vi "RichToFlatnixnet_grpc_EnetFrameRequest.vi"(5 "OutputClusterType":T1, 11 "InputCluster":T4) -> (3 "OutputCluster":T1)   [LabVIEW 2025, in "grpc-xnet_client.lvlib"]
uses:
  grpc-xnet_client.lvlib
  nixnet_grpc_EnetFrameRequest.ctl
  nixnet_grpc_EnetFrameRequest_type_enum/nixnet_grpc_EnetFrameRequest_type_enum.lvclass
  nixnet_grpc_EnetFlags.ctl
  nixnet_grpc_EnetFrameRequest_Flat.ctl
  nixnet_grpc_EnetFrameType.ctl
  nixnet_grpc_EnetFrameRequest_type_enum/nixnet_grpc_EnetFrameRequest_type_enum.lvclass/nixnet_grpc_EnetFrameRequest_type_enum.ctl
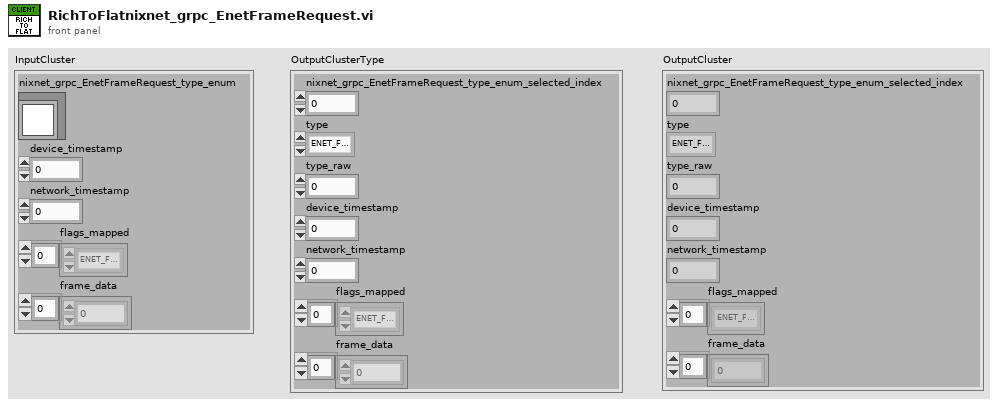
[diagram p1: front panel]
types:
  T1 = typedef "grpc-xnet_client.lvlib/nixnet_grpc_EnetFrameRequest_Flat.ctl" = cluster{"nixnet_grpc_EnetFrameRequest_type_enum_selected_index":i32, "type":T2, "type_raw":u32, "device_timestamp":u64, "network_timestamp":u64, "flags_mapped":T3[], "frame_data":u8[]}
  T2 = typedef "grpc-xnet_client.lvlib/nixnet_grpc_EnetFrameType.ctl" = enum32{"ENET_FRAME_TYPE_DATA", "ENET_FRAME_TYPE_DELAY", "ENET_FRAME_TYPE_FUTURE_TIME_WAIT"}
  T3 = typedef "grpc-xnet_client.lvlib/nixnet_grpc_EnetFlags.ctl" = enum32{"ENET_FLAGS_UNSPECIFIED", "ENET_FLAGS_TRANSMIT", "ENET_FLAGS_RECEIVE", "ENET_FLAGS_NETWORK_SYNCED", "ENET_FLAGS_ERROR"}
  T4 = typedef "grpc-xnet_client.lvlib/nixnet_grpc_EnetFrameRequest.ctl" = cluster{"nixnet_grpc_EnetFrameRequest_type_enum":refnum<class "nixnet_grpc_EnetFrameRequest_type_enum.lvclass">, "device_timestamp":u64, "network_timestamp":u64, "flags_mapped":T3[], "frame_data":u8[]}
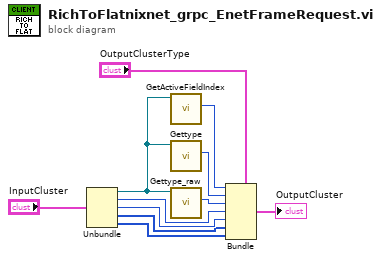
[diagram p0: block diagram]
diagram:
  n1 = Unbundle "Unbundle"("InputCluster") -> ("nixnet_grpc_EnetFrameRequest_type_enum"=w8:refnum<class "nixnet_grpc_EnetFrameRequest_type_enum.lvclass">, "device_timestamp"=w4:u64, "network_timestamp"=w3:u64, "flags_mapped"=w2:T3[], "frame_data"=w1:u8[])
  n2 = call "GetActiveFieldIndex.vi"("OneOfTemplate in"=w8) -> ("Active Field Index"=w7:i32)  [unwired: 8 in, 2 out]
  n3 = call "Gettype.vi"("OneOfTemplate in"=w8) -> ("Get_Val"=w6:T2)  [unwired: 8 in, 2 out]
  n4 = call "Gettype_raw.vi"("OneOfTemplate in"=w8) -> ("Get_Val"=w5:u32)  [unwired: 8 in, 2 out]
  n5 = Bundle "Bundle"(cluster="OutputClusterType", "nixnet_grpc_EnetFrameRequest_type_enum_selected_index"=w7, "type"=w6, "type_raw"=w5, "device_timestamp"=w4, "network_timestamp"=w3, "flags_mapped"=w2, "frame_data"=w1) -> (→"OutputCluster":T1)
